vi "myRIO_TDMS_Builder.vi"(6 "Title":string="IOT Project", 7 "Data":dbl[][](array[numeric]), 8 "error in (no error)":errorcluster, 9 "group name":string="myRIO Data", 11 "Filename.TDMS":path=path "Example Time Domain Data.tdms") -> (0 "error out":errorcluster, 3 "file path out":path)   [LabVIEW 2015]
panel:
  in  "Channel Names":string[](array[string])=["Time Stamp", "Wind Direction", "Wind Speed", "Air Temperature", "Internal Temperature", "Relative Humidity", "Air Pressure", "Rain Accumulation", "Rain Duration", "Rain Intensity", "Hail Duration", "Hail Intensity", "Supply Voltage", "Solar Irradiance"]
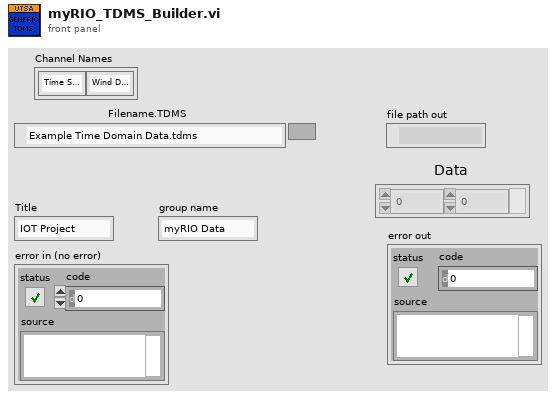
[diagram p1: front panel]
types:
  T1 = enum16{"open", "open or create", "create or replace", "create", "open (read-only)"}
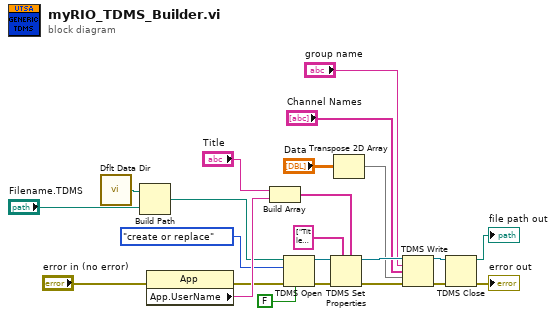
[diagram p0: block diagram]
diagram:
  n1 = call <vilib>:"Dflt Data Dir.vi"() -> ("App:Default Data Directory"=w19:path)
  n2 = Build Path(base path=w19, name or relative path="Filename.TDMS") -> (appended path=w9:path)
  n3 = property class="App"(error in="error in (no error)") -> (error out=w11:errorcluster, "App.UserName"=w15:string)  [unwired: 1 in, 1 out]
  n4 = Build Array("Title", w15) -> (w14:string[])
  n5 = TDMS Open(6:FALSE ("disable buffering (T)"), 8:w11, 10:T1."create or replace" ("operation"), 11:w9) -> (0:w17:errorcluster, 3:w18:refnum<k34>)  [unwired: 3 in]
  n6 = TDMS Set Properties(5:w14, 7:string[] ["Title", "Author"] ("property names"), 8:w17, 11:w18) -> (0:w23:errorcluster, 3:w22:refnum<k34>)  [unwired: 4 out]
  n7 = Transpose 2D Array(2D array="Data") -> (transposed array=w2:dbl[][])
  n8 = TDMS Write(0:w22, 5:"group name", 7:"Channel Names", 9:w2, 11:w23) -> (4:w7:refnum<k34>, 15:w5:errorcluster)  [unwired: 1 in, 2 out]
  n9 = TDMS Close(8:w5, 11:w7) -> (0:→"error out":errorcluster, 3:→"file path out":path)
